vi "Revision Query.vi"(8 "error in (no error)":errorcluster, 11 "VISA resource name":refnum<visa-resource-name>) -> (0 "error out":errorcluster, 1 "Instrument Firmware Revision":string, 2 "Instrument Driver Revision":string, 3 "VISA resource name out":refnum<visa-resource-name>)   [LabVIEW 2021, in "Siglent SDS 1000 2000 Series.lvlib"]
doc: "Queries the current instrument firmware revision and instrument driver revision.\n\nFor detailed driver information including modification history, refer to the <B> Siglent SDS1000 Readme.html </B> file."
uses:
  <instrlib>/Siglent SDS 1000 2000 Series/Siglent SDS 1000 2000 Series.lvlib
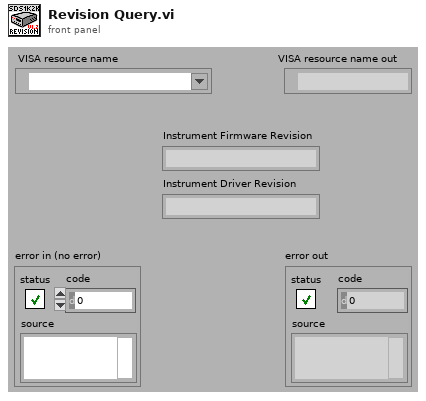
[diagram p1: front panel]
types:
  T1 = cluster{"Major":u16, "Minor":u16, "Fix":u16, "Build":u16}
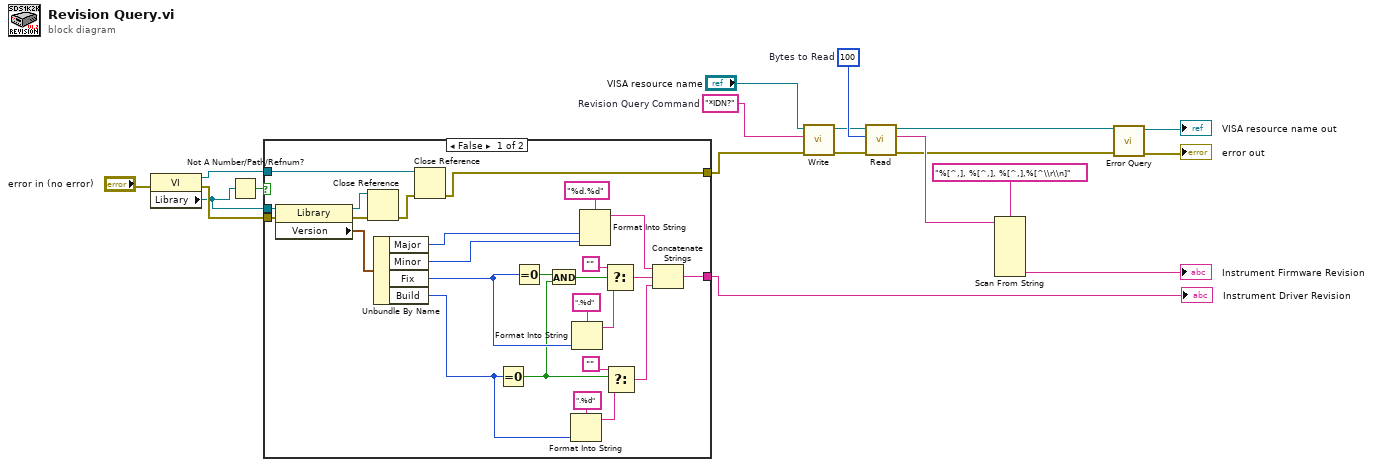
[diagram p0: block diagram]
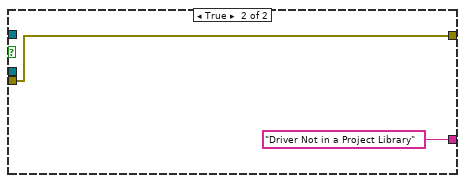
[diagram p2: hidden frame]
diagram:
  w14 = "*IDN?"  # Revision Query Command
  w17 = u32 100  # Bytes to Read
  n1 = property class="VI"(error in="error in (no error)") -> (reference out=w1:refnum<vi>, error out=w4:errorcluster, "Library"=w3:refnum<vi>)  [unwired: 1 in]
  n2 = Not A Number/Path/Refnum?(number/path/refnum=w3) -> (NaN/Path/Refnum?=w2:bool)
  n3 = case shown="False" w2 {
    tunnel: [w24 w46] -> w5
    tunnel: [w23 "Driver Not in a Project Library"] -> w6
    tunnel: w4 -> [w22 w46]
    tunnel: w3 -> [w21 _]
    tunnel: w1 -> [w20 _]
    frame False {
      n4 = property class="Library"(reference=w21, error in=w22) -> (reference out=w44:refnum<vi>, error out=w45:errorcluster, "Version"=w42:T1)
      n5 = Close Reference(reference=w44, error in (no error)=w45) -> (error out=w43:errorcluster)
      n6 = Unbundle By Name(w42) -> ("Major"=w31:u16, "Minor"=w30:u16, "Fix"=w28:u16, "Build"=w29:u16)
      n7 = Close Reference(reference=w20, error in (no error)=w43) -> (error out=w24:errorcluster)
      n8 = Equal To 0?(x=w29) -> (x = 0?=w26:bool)
      n9 = Equal To 0?(x=w28) -> (x = 0?=w27:bool)
      n10 = And(x=w27, y=w26) -> (x .and. y?=w25:bool)
      n11 = Format Into String(format string=".%d", w29) -> (resulting string=w35:string)  [unwired: 2 in, 1 out]
      n12 = Format Into String(format string=".%d", w28) -> (resulting string=w39:string)  [unwired: 2 in, 1 out]
      n13 = Format Into String(format string="%d.%d", w31, w30) -> (resulting string=w37:string)  [unwired: 2 in, 1 out]
      n14 = Select(t="", s=w25, f=w39) -> (s? t:f=w36:string)
      n15 = Select(t="", s=w26, f=w35) -> (s? t:f=w32:string)
      n16 = Concatenate Strings(w37, w36, w32) -> (w23:string)
    }
    frame True {
    }
  }
  "Instrument Driver Revision" <- w6
  n17 = call <instrlib>:"Write.vi"("error in (no error)"=w5, "Write Buffer"=w14, "VISA resource name"="VISA resource name") -> ("error out"=w15:errorcluster, "VISA resource name out"=w16:refnum<visa-resource-name>)  [unwired: 6 in, 1 out]
  n18 = call <instrlib>:"Read.vi"("error in (no error)"=w15, "Byte Count"=w17, "VISA resource name"=w16) -> ("error out"=w10:errorcluster, "Read Buffer"=w13:string, "VISA resource name out"=w11:refnum<visa-resource-name>)  [unwired: 5 in, 1 out]
  n19 = Scan From String(format string="%[^,], %[^,], %[^,],%[^\\r\\n]", input string=w13) -> (output 4=→"Instrument Firmware Revision":string)  [unwired: 9 in, 3 out]
  n20 = call <instrlib>:"Error Query.vi"("error in (no error)"=w10, "VISA resource name"=w11) -> ("error out"=→"error out":errorcluster, "VISA resource name out"=→"VISA resource name out":refnum<visa-resource-name>)  [unwired: 6 in, 2 out]
